vi "myFFT_RowSave.vi"(0 "freqs rows":i32[][](array[numeric]), 1 "小注入模式":u8, 2 "响应模式":u8 max=20, 3 "注入(1号)端口类型":u8(ring) items=["单相", "三相αβ系", "三相同步系", "三相正负序"], 4 "dq同步来源":u8(ring) items=["1号A相", "2号A相"], 5 "index row":i32[](array[numeric]), 6 "采样结果簇":T1, 7 "可用pico数(仅用于模式100)":u16, 9 "f_tick":dbl, 11 "f_mes":i32, 12 "稳态工作点输入":cdb[][](array[numeric]), 13 "写表结果输入":dbl[][](array[numeric]), 14 "基波频率 f_fun":u32=50 min=1 max=100000) -> (10 "稳态工作点输出":cdb[][](array[numeric]), 15 "写表结果输出":dbl[][](array[numeric]))   [LabVIEW 2024]
doc: "对于每个注入循环节，提取出FFT结果中的有效信息，存入稳态寄存器或输出结果寄存器。"
uses:
  <vilib>/Analysis/2dsp.llb/Real FFT.vi
  <vilib>/Analysis/NI_AALPro.lvlib
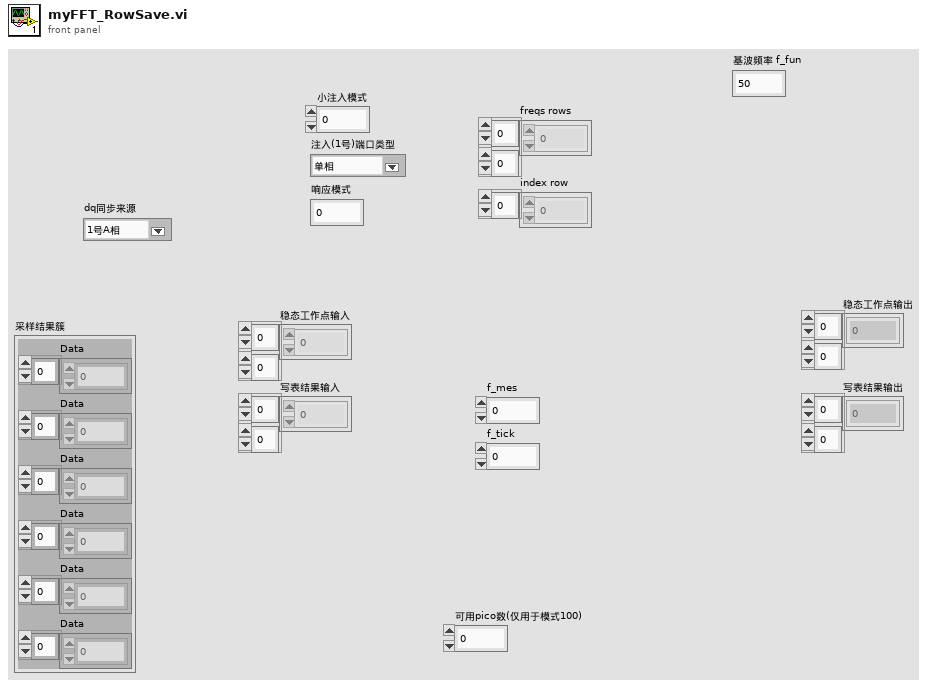
[diagram p1: front panel]
types:
  T1 = cluster{"Data":dbl[], "Data":dbl[], "Data":dbl[], "Data":dbl[], "Data":dbl[], "Data":dbl[]}
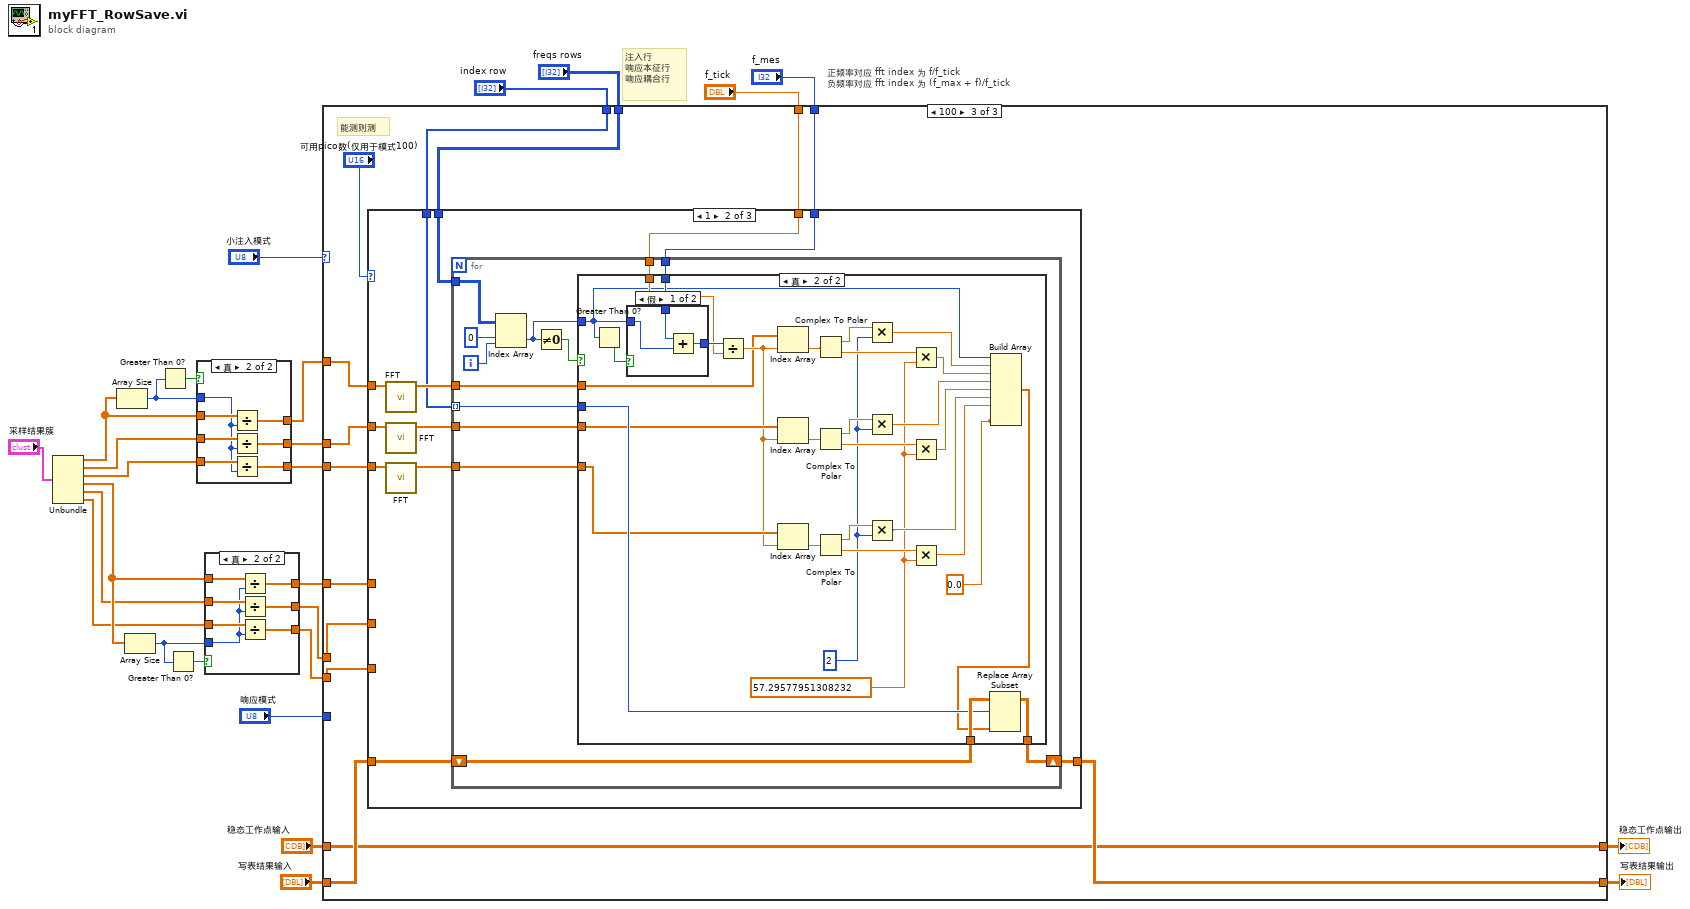
[diagram p0: block diagram]
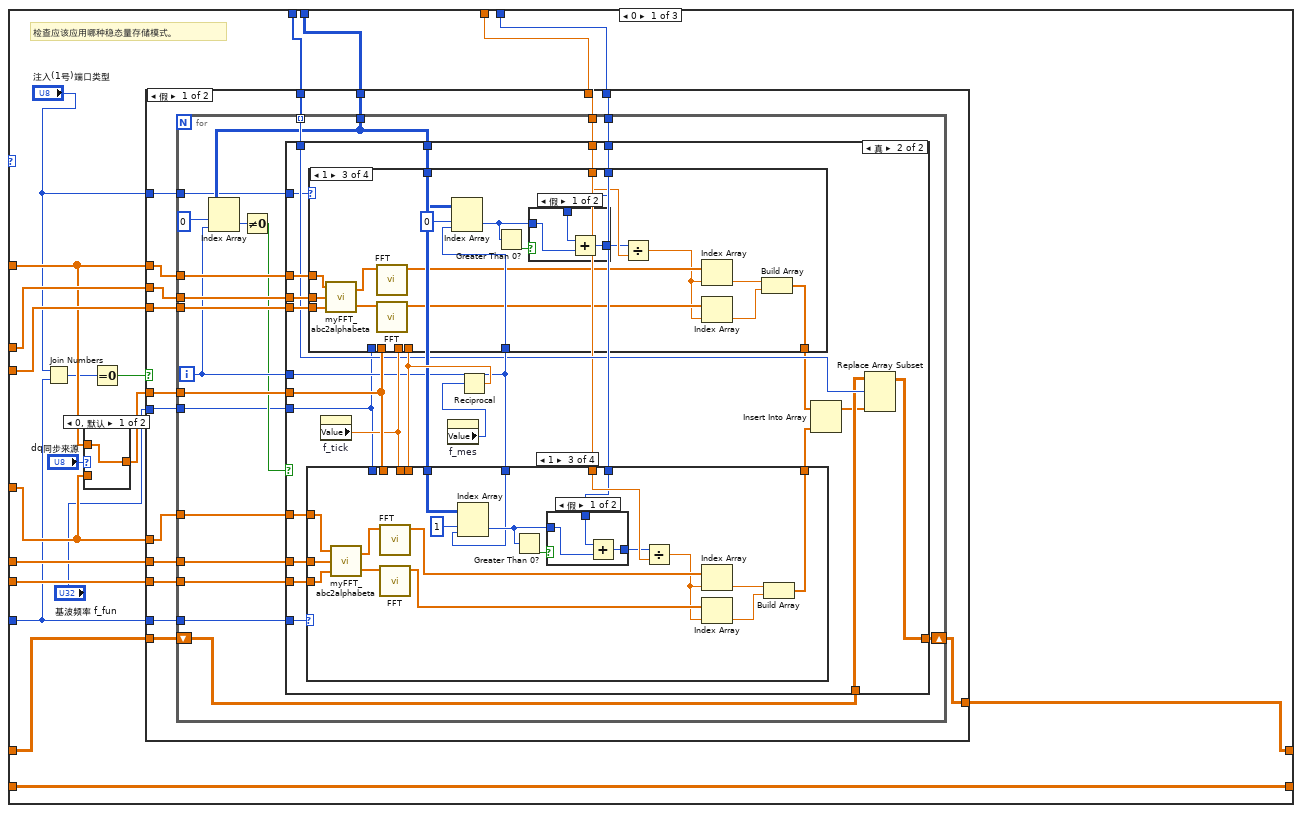
[diagram p4: hidden frame]
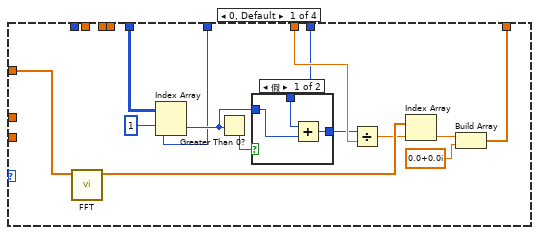
[diagram p7: hidden frame]
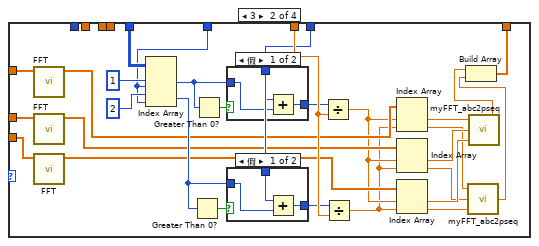
[diagram p9: hidden frame]
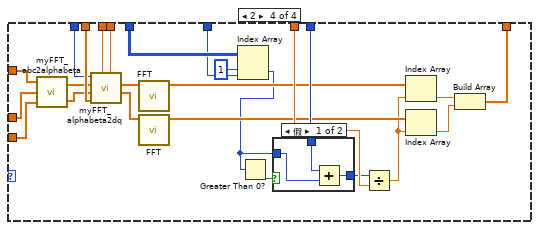
[diagram p13: hidden frame]
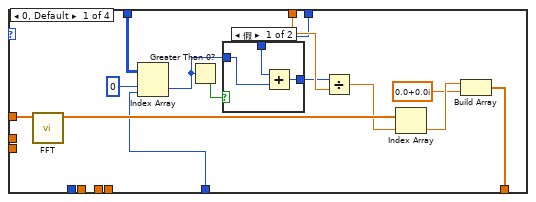
[diagram p15: hidden frame]
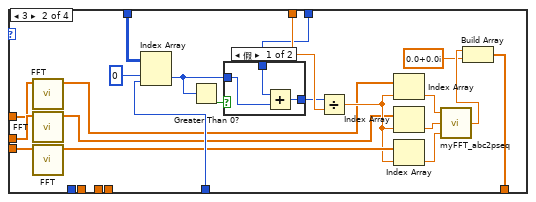
[diagram p17: hidden frame]
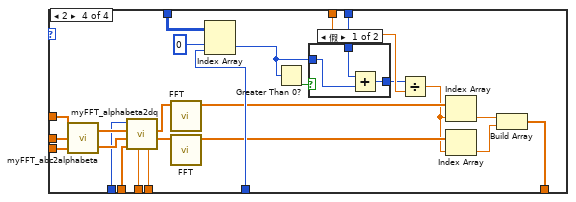
[diagram p20: hidden frame]
diagram:
  # "注入行\n响应本征行\n响应耦合行"
  # "正频率对应 fft index 为 f/f_tick\n负频率对应 fft index 为 (f_max + f)/f_tick"
  n1 = Unbundle("采样结果簇") -> ("Data"=w13:dbl[], "Data"=w11:dbl[], "Data"=w10:dbl[], "Data"=w6:dbl[], "Data"=w5:dbl[], "Data"=w4:dbl[])
  n2 = Array Size(array=w13) -> (size(s)=w16:i32)
  n3 = Array Size(array=w6) -> (size(s)=w7:i32)
  n4 = Greater Than 0?(x=w16) -> (x > 0?=w15:bool)
  n5 = Greater Than 0?(x=w7) -> (x > 0?=w8:bool)
  n6 = case shown="真" w15 {
    tunnel: w16 -> [_ w31]
    tunnel: [w28 w36] -> w14
    tunnel: w13 -> [w28 w37]
    tunnel: [w29 w35] -> w9
    tunnel: [w30 w34] -> w12
    tunnel: w10 -> [w29 w33]
    tunnel: w11 -> [w30 w32]
    frame False {
    }
    frame True {
      n7 = Divide(x=w37, y=w31) -> (x/y=w36:dbl[])
      n8 = Divide(x=w32, y=w31) -> (x/y=w34:dbl[])
      n9 = Divide(x=w33, y=w31) -> (x/y=w35:dbl[])
    }
  }
  n10 = case shown="真" w8 {
    tunnel: w7 -> [_ w41]
    tunnel: [w38 w46] -> w3
    tunnel: w6 -> [w38 w47]
    tunnel: [w39 w45] -> w1
    tunnel: [w40 w44] -> w2
    tunnel: w4 -> [w39 w43]
    tunnel: w5 -> [w40 w42]
    frame False {
    }
    frame True {
      n11 = Divide(x=w47, y=w41) -> (x/y=w46:dbl[])
      n12 = Divide(x=w42, y=w41) -> (x/y=w44:dbl[])
      n13 = Divide(x=w43, y=w41) -> (x/y=w45:dbl[])
    }
  }
  n14 = case shown="100" "小注入模式" {
    tunnel: "写表结果输入" -> [w67 w396 w869]
    tunnel: [w67 w395 w868] -> w24
    tunnel: "稳态工作点输入" -> [w58 w394 w867]
    tunnel: [w54 w394 w867] -> w25
    tunnel: w14 -> [w56 w399 w865]
    tunnel: w12 -> [w62 w404 w864]
    tunnel: w9 -> [w61 w403 w863]
    tunnel: w3 -> [w57 w400 w862]
    tunnel: w2 -> [w60 w402 w861]
    tunnel: w1 -> [w59 w401 w860]
    tunnel: "响应模式" -> [w51 w392 _]
    tunnel: "freqs rows" -> [w64 w406 w857]
    tunnel: "f_tick" -> [w65 w407 w859]
    tunnel: "f_mes" -> [w66 w408 w858]
    tunnel: "index row" -> [w63 w405 w856]
    frame 0 {
      # "检查应该应用哪种稳态量存储模式。"
      n15 = Join Numbers(hi="注入(1号)端口类型", lo=w51) -> ((hi.lo)=w50:u16)
      n16 = case shown="0, 默认" "dq同步来源" {
        tunnel: w56 -> [w68 _]
        tunnel: w57 -> [_ w69]
        tunnel: [w68 w69] -> w55
        frame 0, Default {
        }
        frame 1 {
        }
      }
      n17 = Equal To 0?(x=w50) -> (x = 0?=w49:bool)
      n18 = case shown="假" w49 {
        tunnel: w61 -> [w78 w335]
        tunnel: w56 -> [w81 w343]
        tunnel: "注入(1号)端口类型" -> [w70 _]
        tunnel: w51 -> [w73 _]
        tunnel: w57 -> [w77 _]
        tunnel: w60 -> [w76 _]
        tunnel: w59 -> [w75 _]
        tunnel: w62 -> [w79 w342]
        tunnel: w64 -> [w84 w341]
        tunnel: w58 -> [w80 w338]
        tunnel: w63 -> [w85 w337]
        tunnel: [w71 w336] -> w54
        tunnel: w65 -> [w83 w340]
        tunnel: w66 -> [w82 w339]
        tunnel: w55 -> [w74 _]
        tunnel: "基波频率 f_fun" -> [w72 _]
        frame False {
          n19 = for {
            tunnel: w85 -> [w95] mode=indexing
            tunnel: w84 -> [w91]
            tunnel: w83 -> [w98]
            tunnel: w82 -> [w97]
            tunnel: w81 -> [w105]
            shift-right: [w94] -> w71
            shift-left: w80 -> [w87]
            tunnel: w79 -> [w104]
            tunnel: w78 -> [w103]
            tunnel: w77 -> [w102]
            tunnel: w76 -> [w101]
            tunnel: w75 -> [w100]
            tunnel: w74 -> [w99]
            tunnel: w73 -> [w96]
            tunnel: w72 -> [w88]
            tunnel: w70 -> [w86]
            i -> [w92]
            n20 = Index Array(array=w91, index (row)=0 ("索引"), index (col)=w92) -> (element=w90:i32)
            n21 = Not Equal To 0?(x=w90) -> (x != 0?=w89:bool)
            n22 = case shown="真" w89 {
              tunnel: w105 -> [_ w129]
              tunnel: w104 -> [_ w128]
              tunnel: w103 -> [_ w127]
              tunnel: w102 -> [_ w126]
              tunnel: w101 -> [_ w125]
              tunnel: w100 -> [_ w124]
              tunnel: w99 -> [_ w123]
              tunnel: w91 -> [_ w119]
              tunnel: w98 -> [_ w108]
              tunnel: w97 -> [_ w118]
              tunnel: w92 -> [_ w117]
              tunnel: w96 -> [_ w116]
              tunnel: w95 -> [_ w115]
              tunnel: w87 -> [w106 w114]
              tunnel: [w106 w113] -> w94
              tunnel: w88 -> [_ w109]
              tunnel: w86 -> [_ w107]
              frame False {
              }
              frame True {
                n23 = property on="f_tick" class="DigNum (严格)"() -> ("Value"=w120:dbl)  [unwired: 2 in, 2 out]
                n24 = property on="f_mes" class="DigNum (严格)"() -> ("Value"=w122:i32)  [unwired: 2 in, 2 out]
                n25 = Reciprocal(x=w122) -> (1/x=w121:dbl)
                n26 = case shown="1" w116 {
                  tunnel: w121 -> [_ _ _ w232]
                  tunnel: w120 -> [_ _ _ w231]
                  tunnel: w123 -> [_ _ _ w230]
                  tunnel: w124 -> [_ w171 w200 w227]
                  tunnel: w125 -> [_ w173 w201 w226]
                  tunnel: w126 -> [w140 w174 w202 w225]
                  tunnel: w119 -> [w143 w172 w199 w223]
                  tunnel: w108 -> [w142 w176 w198 w222]
                  tunnel: w118 -> [w141 w175 w197 w221]
                  tunnel: w117 -> [w137 w148 w193 w218]
                  tunnel: [w135 w163 w190 w215] -> w111
                  tunnel: w109 -> [_ _ _ w209]
                  frame 0, Default {
                    n27 = call-poly <vilib>:"FFT.vi"("X"=w140) -> ("FFT {X}"=w136:cdb[])  [unwired: 9 in, 1 out]
                    n28 = Index Array(array=w143, index (row)=1 ("索引"), index (col)=w137) -> (element=w138:i32)
                    n29 = Greater Than 0?(x=w138) -> (x > 0?=w134:bool)
                    n30 = case shown="假" w134 {
                      tunnel: w138 -> [w145 w147]
                      tunnel: w141 -> [w146 _]
                      tunnel: [w144 w147] -> w133
                      frame False {
                        n31 = Add(x=w146, y=w145) -> (x+y=w144:i32)
                      }
                      frame True {
                      }
                    }
                    n32 = Divide(x=w133, y=w142) -> (x/y=w132:dbl)
                    n33 = Index Array(array=w136, index=w132) -> (element=w131:cdb)
                    n34 = Build Array(w131, cdb 0.0+0.0i ("元素")) -> (w135:cdb[])
                  }
                  frame 3 {
                    n35 = call-poly <vilib>:"FFT.vi"("X"=w174) -> ("FFT {X}"=w166:cdb[])  [unwired: 9 in, 1 out]
                    n36 = call-poly <vilib>:"FFT.vi"("X"=w173) -> ("FFT {X}"=w165:cdb[])  [unwired: 9 in, 1 out]
                    n37 = call-poly <vilib>:"FFT.vi"("X"=w171) -> ("FFT {X}"=w164:cdb[])  [unwired: 9 in, 1 out]
                    n38 = Index Array(array=w172, index (row) #1=1 ("索引"), index (col) #1=w148, index (row) #2=2 ("索引 (行)"), index (col) #2=w148) -> (element #1=w169:i32, element #2=w167:i32)
                    n39 = Greater Than 0?(x=w167) -> (x > 0?=w156:bool)
                    n40 = Greater Than 0?(x=w169) -> (x > 0?=w162:bool)
                    n41 = case shown="假" w162 {
                      tunnel: w169 -> [w182 w184]
                      tunnel: w175 -> [w183 _]
                      tunnel: [w181 w184] -> w161
                      frame False {
                        n42 = Add(x=w183, y=w182) -> (x+y=w181:i32)
                      }
                      frame True {
                      }
                    }
                    n43 = case shown="假" w156 {
                      tunnel: w167 -> [w178 w180]
                      tunnel: w175 -> [w179 _]
                      tunnel: [w177 w180] -> w155
                      frame False {
                        n44 = Add(x=w179, y=w178) -> (x+y=w177:i32)
                      }
                      frame True {
                      }
                    }
                    n45 = Divide(x=w161, y=w176) -> (x/y=w160:dbl)
                    n46 = Divide(x=w155, y=w176) -> (x/y=w154:dbl)
                    n47 = Index Array(array=w166, index #1=w160, index #2=w154) -> (element #1=w159:cdb, element #2=w153:cdb)
                    n48 = Index Array(array=w165, index #1=w160, index #2=w154) -> (element #1=w158:cdb, element #2=w152:cdb)
                    n49 = Index Array(array=w164, index #1=w160, index #2=w154) -> (element #1=w157:cdb, element #2=w151:cdb)
                    n50 = call "myFFT_abc2pseq.vi"("C spec"=w151, "B spec"=w152, "A spec"=w153) -> ("p seq spec"=w149:cdb)
                    n51 = call "myFFT_abc2pseq.vi"("C spec"=w157, "B spec"=w158, "A spec"=w159) -> ("p seq spec"=w150:cdb)
                    n52 = Build Array(w150, w149) -> (w163:cdb[])
                  }
                  frame 1 {
                    n53 = call "myFFT_abc2alphabeta.vi"("C wave"=w200, "B wave"=w201, "A wave"=w202) -> ("beta wave"=w196:dbl[], "alpha wave"=w203:dbl[])
                    n54 = call-poly <vilib>:"FFT.vi"("X"=w203) -> ("FFT {X}"=w192:cdb[])  [unwired: 9 in, 1 out]
                    n55 = call-poly <vilib>:"FFT.vi"("X"=w196) -> ("FFT {X}"=w191:cdb[])  [unwired: 9 in, 1 out]
                    n56 = Index Array(array=w199, index (row)=1 ("索引"), index (col)=w193) -> (element=w194:i32)
                    n57 = Greater Than 0?(x=w194) -> (x > 0?=w189:bool)
                    n58 = case shown="假" w189 {
                      tunnel: w194 -> [w205 w207]
                      tunnel: w197 -> [w206 _]
                      tunnel: [w204 w207] -> w188
                      frame False {
                        n59 = Add(x=w206, y=w205) -> (x+y=w204:i32)
                      }
                      frame True {
                      }
                    }
                    n60 = Divide(x=w188, y=w198) -> (x/y=w187:dbl)
                    n61 = Index Array(array=w192, index=w187) -> (element=w186:cdb)
                    n62 = Index Array(array=w191, index=w187) -> (element=w185:cdb)
                    n63 = Build Array(w186, w185) -> (w190:cdb[])
                  }
                  frame 2 {
                    n64 = call "myFFT_abc2alphabeta.vi"("C wave"=w227, "B wave"=w226, "A wave"=w225) -> ("beta wave"=w228:dbl[], "alpha wave"=w229:dbl[])
                    n65 = call "myFFT_alphabeta2dq.vi"("t_tick"=w232, "f_tick"=w231, "ref wave"=w230, "beta wave"=w228, "alpha wave"=w229, "基波频率"=w209) -> ("q wave"=w220:dbl[], "d wave"=w224:dbl[])  [unwired: 4 in]
                    n66 = call-poly <vilib>:"FFT.vi"("X"=w224) -> ("FFT {X}"=w217:cdb[])  [unwired: 9 in, 1 out]
                    n67 = call-poly <vilib>:"FFT.vi"("X"=w220) -> ("FFT {X}"=w216:cdb[])  [unwired: 9 in, 1 out]
                    n68 = Index Array(array=w223, index (row)=1 ("索引"), index (col)=w218) -> (element=w208:i32)
                    n69 = Greater Than 0?(x=w208) -> (x > 0?=w214:bool)
                    n70 = case shown="假" w214 {
                      tunnel: w208 -> [w234 w236]
                      tunnel: w221 -> [w235 _]
                      tunnel: [w233 w236] -> w213
                      frame False {
                        n71 = Add(x=w235, y=w234) -> (x+y=w233:i32)
                      }
                      frame True {
                      }
                    }
                    n72 = Divide(x=w213, y=w222) -> (x/y=w212:dbl)
                    n73 = Index Array(array=w217, index=w212) -> (element=w211:cdb)
                    n74 = Index Array(array=w216, index=w212) -> (element=w210:cdb)
                    n75 = Build Array(w211, w210) -> (w215:cdb[])
                  }
                }
                n76 = case shown="1" w107 {
                  tunnel: w121 -> [_ _ _ w327]
                  tunnel: w120 -> [_ _ _ w326]
                  tunnel: w123 -> [_ _ _ w325]
                  tunnel: w129 -> [w246 w271 w298 w322]
                  tunnel: w119 -> [w250 w275 w293 w318]
                  tunnel: w108 -> [w249 w274 w295 w317]
                  tunnel: w118 -> [w248 w255 w294 w316]
                  tunnel: w128 -> [_ w272 w297 w321]
                  tunnel: w127 -> [_ w273 w296 w320]
                  tunnel: w117 -> [w243 w268 w288 w312]
                  tunnel: [w242 w266 w285 w309] -> w112
                  tunnel: w109 -> [_ _ _ w303]
                  frame 0, Default {
                    n77 = call-poly <vilib>:"FFT.vi"("X"=w246) -> ("FFT {X}"=w247:cdb[])  [unwired: 9 in, 1 out]
                    n78 = Index Array(array=w250, index (row)=0 ("索引"), index (col)=w243) -> (element=w244:i32)
                    n79 = Greater Than 0?(x=w244) -> (x > 0?=w241:bool)
                    n80 = case shown="假" w241 {
                      tunnel: w244 -> [w252 w254]
                      tunnel: w248 -> [w253 _]
                      tunnel: [w251 w254] -> w240
                      frame False {
                        n81 = Add(x=w253, y=w252) -> (x+y=w251:i32)
                      }
                      frame True {
                      }
                    }
                    n82 = Divide(x=w240, y=w249) -> (x/y=w239:dbl)
                    n83 = Index Array(array=w247, index=w239) -> (element=w238:cdb)
                    n84 = Build Array(w238, cdb 0.0+0.0i ("元素")) -> (w242:cdb[])
                  }
                  frame 3 {
                    n85 = call-poly <vilib>:"FFT.vi"("X"=w271) -> ("FFT {X}"=w256:cdb[])  [unwired: 9 in, 1 out]
                    n86 = call-poly <vilib>:"FFT.vi"("X"=w272) -> ("FFT {X}"=w257:cdb[])  [unwired: 9 in, 1 out]
                    n87 = call-poly <vilib>:"FFT.vi"("X"=w273) -> ("FFT {X}"=w267:cdb[])  [unwired: 9 in, 1 out]
                    n88 = Index Array(array=w275, index (row)=0 ("索引"), index (col)=w268) -> (element=w269:i32)
                    n89 = Greater Than 0?(x=w269) -> (x > 0?=w265:bool)
                    n90 = case shown="假" w265 {
                      tunnel: w269 -> [w277 w279]
                      tunnel: w255 -> [w278 _]
                      tunnel: [w276 w279] -> w264
                      frame False {
                        n91 = Add(x=w278, y=w277) -> (x+y=w276:i32)
                      }
                      frame True {
                      }
                    }
                    n92 = Divide(x=w264, y=w274) -> (x/y=w263:dbl)
                    n93 = Index Array(array=w256, index=w263) -> (element=w262:cdb)
                    n94 = Index Array(array=w257, index=w263) -> (element=w261:cdb)
                    n95 = Index Array(array=w267, index=w263) -> (element=w260:cdb)
                    n96 = call "myFFT_abc2pseq.vi"("C spec"=w260, "B spec"=w261, "A spec"=w262) -> ("p seq spec"=w259:cdb)
                    n97 = Build Array(w259, cdb 0.0+0.0i ("元素")) -> (w266:cdb[])
                  }
                  frame 1 {
                    n98 = call "myFFT_abc2alphabeta.vi"("C wave"=w296, "B wave"=w297, "A wave"=w298) -> ("beta wave"=w292:dbl[], "alpha wave"=w291:dbl[])
                    n99 = call-poly <vilib>:"FFT.vi"("X"=w291) -> ("FFT {X}"=w287:cdb[])  [unwired: 9 in, 1 out]
                    n100 = call-poly <vilib>:"FFT.vi"("X"=w292) -> ("FFT {X}"=w286:cdb[])  [unwired: 9 in, 1 out]
                    n101 = Index Array(array=w293, index (row)=0 ("索引"), index (col)=w288) -> (element=w289:i32)
                    n102 = Greater Than 0?(x=w289) -> (x > 0?=w284:bool)
                    n103 = case shown="假" w284 {
                      tunnel: w289 -> [w300 w302]
                      tunnel: w294 -> [w301 _]
                      tunnel: [w299 w302] -> w283
                      frame False {
                        n104 = Add(x=w301, y=w300) -> (x+y=w299:i32)
                      }
                      frame True {
                      }
                    }
                    n105 = Divide(x=w283, y=w295) -> (x/y=w282:dbl)
                    n106 = Index Array(array=w287, index=w282) -> (element=w281:cdb)
                    n107 = Index Array(array=w286, index=w282) -> (element=w280:cdb)
                    n108 = Build Array(w281, w280) -> (w285:cdb[])
                  }
                  frame 2 {
                    n109 = call "myFFT_abc2alphabeta.vi"("C wave"=w320, "B wave"=w321, "A wave"=w322) -> ("beta wave"=w323:dbl[], "alpha wave"=w324:dbl[])
                    n110 = call "myFFT_alphabeta2dq.vi"("t_tick"=w327, "f_tick"=w326, "ref wave"=w325, "beta wave"=w323, "alpha wave"=w324, "基波频率"=w303) -> ("q wave"=w319:dbl[], "d wave"=w315:dbl[])  [unwired: 4 in]
                    n111 = call-poly <vilib>:"FFT.vi"("X"=w315) -> ("FFT {X}"=w311:cdb[])  [unwired: 9 in, 1 out]
                    n112 = call-poly <vilib>:"FFT.vi"("X"=w319) -> ("FFT {X}"=w310:cdb[])  [unwired: 9 in, 1 out]
                    n113 = Index Array(array=w318, index (row)=0 ("索引"), index (col)=w312) -> (element=w313:i32)
                    n114 = Greater Than 0?(x=w313) -> (x > 0?=w308:bool)
                    n115 = case shown="假" w308 {
                      tunnel: w313 -> [w329 w331]
                      tunnel: w316 -> [w330 _]
                      tunnel: [w328 w331] -> w307
                      frame False {
                        n116 = Add(x=w330, y=w329) -> (x+y=w328:i32)
                      }
                      frame True {
                      }
                    }
                    n117 = Divide(x=w307, y=w317) -> (x/y=w306:dbl)
                    n118 = Index Array(array=w311, index=w306) -> (element=w305:cdb)
                    n119 = Index Array(array=w310, index=w306) -> (element=w304:cdb)
                    n120 = Build Array(w305, w304) -> (w309:cdb[])
                  }
                }
                n121 = Insert Into Array(array=w112, new element=w111) -> (w110:cdb[])  [unwired: 1 in]
                n122 = Replace Array Subset(array=w114, new element=w110, index (row)=w115) -> (w113:cdb[][])  [unwired: 1 in]
              }
            }
          }
        }
        frame True {
          n123 = call-poly <vilib>:"FFT.vi"("X"=w343) -> ("FFT {X}"=w334:cdb[])  [unwired: 9 in, 1 out]
          n124 = call-poly <vilib>:"FFT.vi"("X"=w342) -> ("FFT {X}"=w333:cdb[])  [unwired: 9 in, 1 out]
          n125 = call-poly <vilib>:"FFT.vi"("X"=w335) -> ("FFT {X}"=w332:cdb[])  [unwired: 9 in, 1 out]
          n126 = for {
            tunnel: w341 -> [w358]
            tunnel: w340 -> [w352]
            tunnel: w339 -> [w351]
            tunnel: w334 -> [w349]
            tunnel: w333 -> [w348]
            tunnel: w332 -> [w347]
            shift-right: [w344] -> w336
            shift-left: w338 -> [w346]
            tunnel: w337 -> [w345] mode=indexing
            i -> [w357]
            n127 = Index Array(array=w358, index (row) #1=0 ("索引"), index (col) #1=w357, index (row) #2=1 ("索引"), index (col) #2=w357) -> (element #1=w353:i32, element #2=w350:i32)
            n128 = Not Equal To 0?(x=w353) -> (x != 0?=w354:bool)
            n129 = case shown="真" w354 {
              tunnel: w353 -> [_ w379]
              tunnel: w352 -> [_ w374]
              tunnel: w351 -> [_ w375]
              tunnel: w350 -> [_ w376]
              tunnel: w349 -> [_ w372]
              tunnel: w348 -> [_ w371]
              tunnel: w347 -> [_ w370]
              tunnel: w346 -> [w359 w365]
              tunnel: w345 -> [_ w364]
              tunnel: [w359 w363] -> w344
              frame False {
              }
              frame True {
                n130 = Greater Than 0?(x=w376) -> (x > 0?=w377:bool)
                n131 = Greater Than 0?(x=w379) -> (x > 0?=w380:bool)
                n132 = case shown="假" w380 {
                  tunnel: w379 -> [w386 w388]
                  tunnel: w375 -> [w387 _]
                  tunnel: [w385 w388] -> w378
                  frame False {
                    n133 = Add(x=w387, y=w386) -> (x+y=w385:i32)
                  }
                  frame True {
                  }
                }
                n134 = case shown="假" w377 {
                  tunnel: w376 -> [w382 w384]
                  tunnel: w375 -> [w383 _]
                  tunnel: [w381 w384] -> w373
                  frame False {
                    n135 = Add(x=w383, y=w382) -> (x+y=w381:i32)
                  }
                  frame True {
                  }
                }
                n136 = Divide(x=w378, y=w374) -> (x/y=w369:dbl)
                n137 = Divide(x=w373, y=w374) -> (x/y=w368:dbl)
                n138 = Index Array(array=w372, index=w369) -> (element=w367:cdb)
                n139 = Index Array(array=w371, index=w368) -> (element=w362:cdb)
                n140 = Index Array(array=w370, index=w368) -> (element=w361:cdb)
                n141 = Build Array(w367, cdb 0.0+0.0i ("元素"), w362, w361) -> (w366:cdb[])
                n142 = Replace Array Subset(array=w365, new element=w366, index (row)=w364) -> (w363:cdb[][])  [unwired: 1 in]
              }
            }
          }
        }
      }
    }
    frame 1, Default {
      # "注入-响应 在小信号测量情况下。在此情况下，对注入输出模式分别做判断。"
      n143 = property on="注入(1号)端口类型" class="Ring (严格)"() -> ("Value"=w393:u8)  [unwired: 2 in, 2 out]
      n144 = Join Numbers(hi=w393, lo=w392) -> ((hi.lo)=w391:u16)
      n145 = property on="dq同步来源" class="Ring (严格)"() -> ("Value"=w389:u8)  [unwired: 2 in, 2 out]
      n146 = property on="基波频率 f_fun" class="DigNum (严格)"() -> ("Value"=w397:u32)  [unwired: 2 in, 2 out]
      n147 = case shown="0, 默认" w389 {
        tunnel: w399 -> [w409 _]
        tunnel: w400 -> [_ w410]
        tunnel: [w409 w410] -> w398
        frame 0, Default {
        }
        frame 1 {
        }
      }
      n148 = Equal To 0?(x=w391) -> (x = 0?=w390:bool)
      n149 = case shown="假" w390 {
        tunnel: w403 -> [w420 w782]
        tunnel: w399 -> [w423 w790]
        tunnel: w393 -> [w412 _]
        tunnel: w392 -> [w415 _]
        tunnel: w400 -> [w419 _]
        tunnel: w402 -> [w418 _]
        tunnel: w401 -> [w417 _]
        tunnel: w404 -> [w421 w789]
        tunnel: w406 -> [w426 w788]
        tunnel: w396 -> [w422 w785]
        tunnel: w405 -> [w427 w784]
        tunnel: [w413 w783] -> w395
        tunnel: w407 -> [w425 w787]
        tunnel: w408 -> [w424 w786]
        tunnel: w398 -> [w416 _]
        tunnel: w397 -> [w414 _]
        tunnel: w394 -> [w411 w778]
        frame False {
          n150 = for {
            tunnel: w427 -> [w439] mode=indexing
            tunnel: w426 -> [w436]
            tunnel: w425 -> [w442]
            tunnel: w424 -> [w441]
            tunnel: w423 -> [w449]
            shift-right: [w438] -> w413
            shift-left: w422 -> [w431]
            tunnel: w421 -> [w448]
            tunnel: w420 -> [w447]
            tunnel: w419 -> [w446]
            tunnel: w418 -> [w445]
            tunnel: w417 -> [w444]
            tunnel: w416 -> [w443]
            tunnel: w415 -> [w440]
            tunnel: w414 -> [w433]
            tunnel: w412 -> [w432]
            tunnel: w411 -> [w430]
            i -> [w428]
            n151 = Index Array(array=w436, index (row)=0 ("索引"), index (col)=w428) -> (element=w435:i32)
            n152 = Index Array(array=w430, index (row)=w428) -> (element=w429:cdb[])  [unwired: 1 in]
            n153 = Not Equal To 0?(x=w435) -> (x != 0?=w434:bool)
            n154 = case shown="真" w434 {
              tunnel: w449 -> [_ w488]
              tunnel: w448 -> [_ w487]
              tunnel: w447 -> [_ w486]
              tunnel: w446 -> [_ w485]
              tunnel: w445 -> [_ w484]
              tunnel: w444 -> [_ w483]
              tunnel: w443 -> [_ w482]
              tunnel: w436 -> [_ w451]
              tunnel: w442 -> [_ w474]
              tunnel: w441 -> [_ w478]
              tunnel: w428 -> [_ w453]
              tunnel: w440 -> [_ w477]
              tunnel: w439 -> [_ w462]
              tunnel: [w450 w476] -> w438
              tunnel: w433 -> [_ w475]
              tunnel: w432 -> [_ w473]
              tunnel: w431 -> [w450 w472]
              tunnel: w429 -> [_ w471]
              frame False {
              }
              frame True {
                n155 = property on="f_tick" class="DigNum (严格)"() -> ("Value"=w479:dbl)  [unwired: 2 in, 2 out]
                n156 = property on="f_mes" class="DigNum (严格)"() -> ("Value"=w481:i32)  [unwired: 2 in, 2 out]
                n157 = Reciprocal(x=w481) -> (1/x=w480:dbl)
                n158 = Index Array(array=w471, index #1=0 ("索引"), index #2=1 ("索引"), index #3=2 ("索引"), index #4=3 ("索引")) -> (element #1=w466:cdb, element #2=w465:cdb, element #3=w464:cdb, element #4=w463:cdb)
                n159 = case shown="0, 默认" w477 {
                  tunnel: w480 -> [_ _ _ w670]
                  tunnel: w479 -> [_ _ _ w669]
                  tunnel: w482 -> [_ _ _ w668]
                  tunnel: w483 -> [_ w603 w635 w665]
                  tunnel: w484 -> [_ w605 w636 w664]
                  tunnel: w485 -> [w569 w606 w637 w663]
                  tunnel: w451 -> [w572 w604 w634 w661]
                  tunnel: w474 -> [w571 w608 w633 w660]
                  tunnel: w478 -> [w570 w607 w632 w659]
                  tunnel: w453 -> [w566 w583 w628 w656]
                  tunnel: w475 -> [_ _ _ w650]
                  tunnel: w464 -> [w560 w581 w620 w646]
                  tunnel: w463 -> [_ w577 w619 w645]
                  tunnel: [w559 w578 w618 w643] -> w459
                  tunnel: [cdb 0.0+0.0i ("元素") w579 w617 w644] -> w458
                  frame 0, Default {
                    n160 = call-poly <vilib>:"FFT.vi"("X"=w569) -> ("FFT {X}"=w565:cdb[])  [unwired: 9 in, 1 out]
                    n161 = Index Array(array=w572, index (row)=1 ("索引"), index (col)=w566) -> (element=w567:i32)
                    n162 = Greater Than 0?(x=w567) -> (x > 0?=w564:bool)
                    n163 = case shown="假" w564 {
                      tunnel: w567 -> [w574 w576]
                      tunnel: w570 -> [w575 _]
                      tunnel: [w573 w576] -> w563
                      frame False {
                        n164 = Add(x=w575, y=w574) -> (x+y=w573:i32)
                      }
                      frame True {
                      }
                    }
                    n165 = Divide(x=w563, y=w571) -> (x/y=w562:dbl)
                    n166 = Index Array(array=w565, index=w562) -> (element=w561:cdb)
                    n167 = Subtract(x=w561, y=w560) -> (x-y=w559:cdb)
                  }
                  frame 3 {
                    n168 = call-poly <vilib>:"FFT.vi"("X"=w606) -> ("FFT {X}"=w598:cdb[])  [unwired: 9 in, 1 out]
                    n169 = call-poly <vilib>:"FFT.vi"("X"=w605) -> ("FFT {X}"=w597:cdb[])  [unwired: 9 in, 1 out]
                    n170 = call-poly <vilib>:"FFT.vi"("X"=w603) -> ("FFT {X}"=w596:cdb[])  [unwired: 9 in, 1 out]
                    n171 = Index Array(array=w604, index (row) #1=1 ("索引"), index (col) #1=w583, index (row) #2=2 ("索引 (行)"), index (col) #2=w583) -> (element #1=w601:i32, element #2=w599:i32)
                    n172 = Greater Than 0?(x=w599) -> (x > 0?=w589:bool)
                    n173 = Greater Than 0?(x=w601) -> (x > 0?=w595:bool)
                    n174 = case shown="假" w595 {
                      tunnel: w601 -> [w614 w616]
                      tunnel: w607 -> [w615 _]
                      tunnel: [w613 w616] -> w594
                      frame False {
                        n175 = Add(x=w615, y=w614) -> (x+y=w613:i32)
                      }
                      frame True {
                      }
                    }
                    n176 = case shown="假" w589 {
                      tunnel: w599 -> [w610 w612]
                      tunnel: w607 -> [w611 _]
                      tunnel: [w609 w612] -> w588
                      frame False {
                        n177 = Add(x=w611, y=w610) -> (x+y=w609:i32)
                      }
                      frame True {
                      }
                    }
                    n178 = Divide(x=w594, y=w608) -> (x/y=w593:dbl)
                    n179 = Divide(x=w588, y=w608) -> (x/y=w587:dbl)
                    n180 = Index Array(array=w598, index #1=w593, index #2=w587) -> (element #1=w592:cdb, element #2=w586:cdb)
                    n181 = Index Array(array=w597, index #1=w593, index #2=w587) -> (element #1=w591:cdb, element #2=w585:cdb)
                    n182 = Index Array(array=w596, index #1=w593, index #2=w587) -> (element #1=w590:cdb, element #2=w584:cdb)
                    n183 = call "myFFT_abc2pseq.vi"("C spec"=w584, "B spec"=w585, "A spec"=w586) -> ("p seq spec"=w580:cdb)
                    n184 = call "myFFT_abc2pseq.vi"("C spec"=w590, "B spec"=w591, "A spec"=w592) -> ("p seq spec"=w582:cdb)
                    n185 = Subtract(x=w582, y=w581) -> (x-y=w578:cdb)
                    n186 = Subtract(x=w580, y=w577) -> (x-y=w579:cdb)
                  }
                  frame 1 {
                    n187 = call "myFFT_abc2alphabeta.vi"("C wave"=w635, "B wave"=w636, "A wave"=w637) -> ("beta wave"=w631:dbl[], "alpha wave"=w638:dbl[])
                    n188 = call-poly <vilib>:"FFT.vi"("X"=w638) -> ("FFT {X}"=w627:cdb[])  [unwired: 9 in, 1 out]
                    n189 = call-poly <vilib>:"FFT.vi"("X"=w631) -> ("FFT {X}"=w626:cdb[])  [unwired: 9 in, 1 out]
                    n190 = Index Array(array=w634, index (row)=1 ("索引"), index (col)=w628) -> (element=w629:i32)
                    n191 = Greater Than 0?(x=w629) -> (x > 0?=w625:bool)
                    n192 = case shown="假" w625 {
                      tunnel: w629 -> [w640 w642]
                      tunnel: w632 -> [w641 _]
                      tunnel: [w639 w642] -> w624
                      frame False {
                        n193 = Add(x=w641, y=w640) -> (x+y=w639:i32)
                      }
                      frame True {
                      }
                    }
                    n194 = Divide(x=w624, y=w633) -> (x/y=w623:dbl)
                    n195 = Index Array(array=w627, index=w623) -> (element=w622:cdb)
                    n196 = Index Array(array=w626, index=w623) -> (element=w621:cdb)
                    n197 = Subtract(x=w622, y=w620) -> (x-y=w618:cdb)
                    n198 = Subtract(x=w621, y=w619) -> (x-y=w617:cdb)
                  }
                  frame 2 {
                    n199 = call "myFFT_abc2alphabeta.vi"("C wave"=w665, "B wave"=w664, "A wave"=w663) -> ("beta wave"=w666:dbl[], "alpha wave"=w667:dbl[])
                    n200 = call "myFFT_alphabeta2dq.vi"("t_tick"=w670, "f_tick"=w669, "ref wave"=w668, "beta wave"=w666, "alpha wave"=w667, "基波频率"=w650) -> ("q wave"=w658:dbl[], "d wave"=w662:dbl[])  [unwired: 4 in]
                    n201 = call-poly <vilib>:"FFT.vi"("X"=w662) -> ("FFT {X}"=w655:cdb[])  [unwired: 9 in, 1 out]
                    n202 = call-poly <vilib>:"FFT.vi"("X"=w658) -> ("FFT {X}"=w654:cdb[])  [unwired: 9 in, 1 out]
                    n203 = Index Array(array=w661, index (row)=1 ("索引"), index (col)=w656) -> (element=w649:i32)
                    n204 = Greater Than 0?(x=w649) -> (x > 0?=w653:bool)
                    n205 = case shown="假" w653 {
                      tunnel: w649 -> [w672 w674]
                      tunnel: w659 -> [w673 _]
                      tunnel: [w671 w674] -> w652
                      frame False {
                        n206 = Add(x=w673, y=w672) -> (x+y=w671:i32)
                      }
                      frame True {
                      }
                    }
                    n207 = Divide(x=w652, y=w660) -> (x/y=w651:dbl)
                    n208 = Index Array(array=w655, index=w651) -> (element=w648:cdb)
                    n209 = Index Array(array=w654, index=w651) -> (element=w647:cdb)
                    n210 = Subtract(x=w648, y=w646) -> (x-y=w643:cdb)
                    n211 = Subtract(x=w647, y=w645) -> (x-y=w644:cdb)
                  }
                }
                n212 = case shown="2" w473 {
                  tunnel: w480 -> [_ _ _ w773]
                  tunnel: w479 -> [_ _ _ w772]
                  tunnel: w482 -> [_ _ _ w771]
                  tunnel: w488 -> [w685 w711 w741 w768]
                  tunnel: w451 -> [w689 w715 w736 w764]
                  tunnel: w474 -> [w688 w714 w738 w763]
                  tunnel: w478 -> [w687 w698 w737 w762]
                  tunnel: w487 -> [_ w712 w740 w767]
                  tunnel: w486 -> [_ w713 w739 w766]
                  tunnel: w453 -> [w682 w708 w731 w758]
                  tunnel: w475 -> [_ _ _ w752]
                  tunnel: w466 -> [w677 w696 w723 w748]
                  tunnel: w465 -> [_ _ w722 w749]
                  tunnel: [cdb 0.0+0.0i ("元素") cdb 0.0+0.0i ("元素") w721 w746] -> w461
                  tunnel: [w675 w695 w720 w747] -> w460
                  frame 0, Default {
                    n213 = call-poly <vilib>:"FFT.vi"("X"=w685) -> ("FFT {X}"=w686:cdb[])  [unwired: 9 in, 1 out]
                    n214 = Index Array(array=w689, index (row)=0 ("索引"), index (col)=w682) -> (element=w683:i32)
                    n215 = Greater Than 0?(x=w683) -> (x > 0?=w681:bool)
                    n216 = case shown="假" w681 {
                      tunnel: w683 -> [w691 w693]
                      tunnel: w687 -> [w692 _]
                      tunnel: [w690 w693] -> w680
                      frame False {
                        n217 = Add(x=w692, y=w691) -> (x+y=w690:i32)
                      }
                      frame True {
                      }
                    }
                    n218 = Divide(x=w680, y=w688) -> (x/y=w679:dbl)
                    n219 = Index Array(array=w686, index=w679) -> (element=w678:cdb)
                    n220 = Subtract(x=w678, y=w677) -> (x-y=w675:cdb)
                  }
                  frame 3 {
                    n221 = call-poly <vilib>:"FFT.vi"("X"=w711) -> ("FFT {X}"=w699:cdb[])  [unwired: 9 in, 1 out]
                    n222 = call-poly <vilib>:"FFT.vi"("X"=w712) -> ("FFT {X}"=w700:cdb[])  [unwired: 9 in, 1 out]
                    n223 = call-poly <vilib>:"FFT.vi"("X"=w713) -> ("FFT {X}"=w707:cdb[])  [unwired: 9 in, 1 out]
                    n224 = Index Array(array=w715, index (row)=0 ("索引"), index (col)=w708) -> (element=w709:i32)
                    n225 = Greater Than 0?(x=w709) -> (x > 0?=w706:bool)
                    n226 = case shown="假" w706 {
                      tunnel: w709 -> [w717 w719]
                      tunnel: w698 -> [w718 _]
                      tunnel: [w716 w719] -> w705
                      frame False {
                        n227 = Add(x=w718, y=w717) -> (x+y=w716:i32)
                      }
                      frame True {
                      }
                    }
                    n228 = Divide(x=w705, y=w714) -> (x/y=w704:dbl)
                    n229 = Index Array(array=w699, index=w704) -> (element=w703:cdb)
                    n230 = Index Array(array=w700, index=w704) -> (element=w702:cdb)
                    n231 = Index Array(array=w707, index=w704) -> (element=w701:cdb)
                    n232 = call "myFFT_abc2pseq.vi"("C spec"=w701, "B spec"=w702, "A spec"=w703) -> ("p seq spec"=w697:cdb)
                    n233 = Subtract(x=w697, y=w696) -> (x-y=w695:cdb)
                  }
                  frame 1 {
                    n234 = call "myFFT_abc2alphabeta.vi"("C wave"=w739, "B wave"=w740, "A wave"=w741) -> ("beta wave"=w735:dbl[], "alpha wave"=w734:dbl[])
                    n235 = call-poly <vilib>:"FFT.vi"("X"=w734) -> ("FFT {X}"=w730:cdb[])  [unwired: 9 in, 1 out]
                    n236 = call-poly <vilib>:"FFT.vi"("X"=w735) -> ("FFT {X}"=w729:cdb[])  [unwired: 9 in, 1 out]
                    n237 = Index Array(array=w736, index (row)=0 ("索引"), index (col)=w731) -> (element=w732:i32)
                    n238 = Greater Than 0?(x=w732) -> (x > 0?=w728:bool)
                    n239 = case shown="假" w728 {
                      tunnel: w732 -> [w743 w745]
                      tunnel: w737 -> [w744 _]
                      tunnel: [w742 w745] -> w727
                      frame False {
                        n240 = Add(x=w744, y=w743) -> (x+y=w742:i32)
                      }
                      frame True {
                      }
                    }
                    n241 = Divide(x=w727, y=w738) -> (x/y=w726:dbl)
                    n242 = Index Array(array=w730, index=w726) -> (element=w725:cdb)
                    n243 = Index Array(array=w729, index=w726) -> (element=w724:cdb)
                    n244 = Subtract(x=w725, y=w723) -> (x-y=w720:cdb)
                    n245 = Subtract(x=w724, y=w722) -> (x-y=w721:cdb)
                  }
                  frame 2 {
                    n246 = call "myFFT_abc2alphabeta.vi"("C wave"=w766, "B wave"=w767, "A wave"=w768) -> ("beta wave"=w769:dbl[], "alpha wave"=w770:dbl[])
                    n247 = call "myFFT_alphabeta2dq.vi"("t_tick"=w773, "f_tick"=w772, "ref wave"=w771, "beta wave"=w769, "alpha wave"=w770, "基波频率"=w752) -> ("q wave"=w765:dbl[], "d wave"=w761:dbl[])  [unwired: 4 in]
                    n248 = call-poly <vilib>:"FFT.vi"("X"=w761) -> ("FFT {X}"=w757:cdb[])  [unwired: 9 in, 1 out]
                    n249 = call-poly <vilib>:"FFT.vi"("X"=w765) -> ("FFT {X}"=w756:cdb[])  [unwired: 9 in, 1 out]
                    n250 = Index Array(array=w764, index (row)=0 ("索引"), index (col)=w758) -> (element=w759:i32)
                    n251 = Greater Than 0?(x=w759) -> (x > 0?=w755:bool)
                    n252 = case shown="假" w755 {
                      tunnel: w759 -> [w775 w777]
                      tunnel: w762 -> [w776 _]
                      tunnel: [w774 w777] -> w754
                      frame False {
                        n253 = Add(x=w776, y=w775) -> (x+y=w774:i32)
                      }
                      frame True {
                      }
                    }
                    n254 = Divide(x=w754, y=w763) -> (x/y=w753:dbl)
                    n255 = Index Array(array=w757, index=w753) -> (element=w751:cdb)
                    n256 = Index Array(array=w756, index=w753) -> (element=w750:cdb)
                    n257 = Subtract(x=w751, y=w748) -> (x-y=w747:cdb)
                    n258 = Subtract(x=w750, y=w749) -> (x-y=w746:cdb)
                  }
                }
                n259 = property on="小注入模式" class="DigNum (严格)"() -> ("Value"=w456:u8)  [unwired: 2 in, 2 out]
                n260 = property on="响应模式" class="DigNum (严格)"() -> ("Value"=w457:u8)  [unwired: 2 in, 2 out]
                n261 = Join Numbers(hi=w456, lo=w457) -> ((hi.lo)=w455:u16)
                n262 = Index Array(array=w451, index (row)=0 ("索引"), index (col)=w453) -> (element=w452:i32)
                n263 = case shown="769..771, 1281..1283" w455 {
                  tunnel: [w489 w504 w526 w527 w539] -> w476
                  tunnel: w472 -> [w489 w503 w525 w528 w540]
                  tunnel: w462 -> [_ w496 w515 w529 w541]
                  tunnel: w461 -> [_ _ _ w534 w550]
                  tunnel: w460 -> [_ w499 w519 _ _]
                  tunnel: w459 -> [_ w498 w518 w535 w552]
                  tunnel: w458 -> [_ _ w517 _ w551]
                  tunnel: w452 -> [_ w490 w505 _ _]
                  frame 0, Default {
                  }
                  frame 256, 512, 1024, 1536 {
                    # "自轴注入，自轴响应"
                    n264 = Divide(x=w498, y=w499) -> (x/y=w502:cdb)
                    n265 = Complex To Polar(r * e^(i*theta)=w502) -> (r=w493:dbl, theta=w501:dbl)
                    n266 = To Double Precision Float(number=w490) -> (double precision float=w491:dbl)
                    n267 = Multiply(x=w501, y=57.29577951308232) -> (x*y=w492:dbl)
                    n268 = Replace Array Subset(array=w503, new element #1=w491, index (row) #1=w496, index (col) #1=0, new element #2=w493, index (row) #2=w496, index (col) #2=1, new element #3=w492, index (row) #3=w496, index (col) #3=2) -> (w504:dbl[][])
                  }
                  frame 257..259, 513..515, 1025..1027, 1537..1539 {
                    w520 = 57.29577951308232
                    # "自轴注入，自、互轴响应"
                    n269 = Divide(x=w518, y=w519) -> (x/y=w524:cdb)
                    n270 = Divide(x=w517, y=w519) -> (x/y=w521:cdb)
                    n271 = Complex To Polar(r * e^(i*theta)=w524) -> (r=w510:dbl, theta=w523:dbl)
                    n272 = Complex To Polar(r * e^(i*theta)=w521) -> (r=w509:dbl, theta=w522:dbl)
                    n273 = To Double Precision Float(number=w505) -> (double precision float=w506:dbl)
                    n274 = Multiply(x=w523, y=w520) -> (x*y=w507:dbl)
                    n275 = Multiply(x=w522, y=w520) -> (x*y=w508:dbl)
                    n276 = Replace Array Subset(array=w525, new element #1=w506, index (row) #1=w515, index (col) #1=0, new element #2=w510, index (row) #2=w515, index (col) #2=1, new element #3=w507, index (row) #3=w515, index (col) #3=2, new element #4=w509, index (row) #4=w515, index (col) #4=3, new element #5=w508, index (row) #5=w515, index (col) #5=4) -> (w526:dbl[][])
                  }
                  frame 768, 1280 {
                    # "互轴注入，自轴响应"
                    n277 = Divide(x=w535, y=w534) -> (x/y=w538:cdb)
                    n278 = Complex To Polar(r * e^(i*theta)=w538) -> (r=w531:dbl, theta=w537:dbl)
                    n279 = Multiply(x=w537, y=57.29577951308232) -> (x*y=w533:dbl)
                    n280 = Replace Array Subset(array=w528, new element #1=w531, index (row) #1=w529, index (col) #1=5, new element #2=w533, index (row) #2=w529, index (col) #2=6) -> (w527:dbl[][])
                  }
                  frame 769..771, 1281..1283 {
                    w553 = 57.29577951308232
                    # "互轴注入，自、互轴响应"
                    n281 = Divide(x=w552, y=w550) -> (x/y=w557:cdb)
                    n282 = Divide(x=w551, y=w550) -> (x/y=w554:cdb)
                    n283 = Complex To Polar(r * e^(i*theta)=w557) -> (r=w543:dbl, theta=w556:dbl)
                    n284 = Complex To Polar(r * e^(i*theta)=w554) -> (r=w547:dbl, theta=w555:dbl)
                    n285 = Multiply(x=w556, y=w553) -> (x*y=w545:dbl)
                    n286 = Multiply(x=w555, y=w553) -> (x*y=w549:dbl)
                    n287 = Replace Array Subset(array=w540, new element #1=w543, index (row) #1=w541, index (col) #1=5, new element #2=w545, index (row) #2=w541, index (col) #2=6, new element #3=w547, index (row) #3=w541, index (col) #3=7, new element #4=w549, index (row) #4=w541, index (col) #4=8) -> (w539:dbl[][])
                  }
                }
              }
            }
          }
        }
        frame True {
          n288 = call-poly <vilib>:"FFT.vi"("X"=w790) -> ("FFT {X}"=w781:cdb[])  [unwired: 9 in, 1 out]
          n289 = call-poly <vilib>:"FFT.vi"("X"=w789) -> ("FFT {X}"=w780:cdb[])  [unwired: 9 in, 1 out]
          n290 = call-poly <vilib>:"FFT.vi"("X"=w782) -> ("FFT {X}"=w779:cdb[])  [unwired: 9 in, 1 out]
          n291 = for {
            tunnel: w788 -> [w807]
            tunnel: w787 -> [w802]
            tunnel: w786 -> [w801]
            tunnel: w781 -> [w799]
            tunnel: w780 -> [w798]
            tunnel: w779 -> [w797]
            shift-right: [w794] -> w783
            shift-left: w785 -> [w796]
            tunnel: w784 -> [w795] mode=indexing
            tunnel: w778 -> [w793]
            i -> [w792]
            n292 = Index Array(array=w807, index (row) #1=0 ("索引"), index (col) #1=w792, index (row) #2=1 ("索引"), index (col) #2=w792) -> (element #1=w803:i32, element #2=w800:i32)
            n293 = Index Array(array=w793, index (row)=w792) -> (element=w791:cdb[])  [unwired: 1 in]
            n294 = Not Equal To 0?(x=w803) -> (x != 0?=w804:bool)
            n295 = case shown="真" w804 {
              tunnel: w803 -> [_ w809]
              tunnel: w802 -> [_ w842]
              tunnel: w801 -> [_ w843]
              tunnel: w800 -> [_ w844]
              tunnel: w799 -> [_ w840]
              tunnel: w798 -> [_ w839]
              tunnel: w797 -> [_ w838]
              tunnel: w796 -> [w808 w835]
              tunnel: w795 -> [_ w834]
              tunnel: [w808 w833] -> w794
              tunnel: w791 -> [_ w831]
              frame False {
              }
              frame True {
                w815 = 57.29577951308232
                n296 = Greater Than 0?(x=w844) -> (x > 0?=w845:bool)
                n297 = Greater Than 0?(x=w809) -> (x > 0?=w847:bool)
                n298 = case shown="假" w847 {
                  tunnel: w809 -> [w853 w855]
                  tunnel: w843 -> [w854 _]
                  tunnel: [w852 w855] -> w846
                  frame False {
                    n299 = Add(x=w854, y=w853) -> (x+y=w852:i32)
                  }
                  frame True {
                  }
                }
                n300 = case shown="假" w845 {
                  tunnel: w844 -> [w849 w851]
                  tunnel: w843 -> [w850 _]
                  tunnel: [w848 w851] -> w841
                  frame False {
                    n301 = Add(x=w850, y=w849) -> (x+y=w848:i32)
                  }
                  frame True {
                  }
                }
                n302 = Index Array(array=w831, index #1=0 ("索引"), index #2=2 ("索引"), index #3=3 ("索引")) -> (element #1=w829:cdb, element #2=w823:cdb, element #3=w824:cdb)
                n303 = Divide(x=w846, y=w842) -> (x/y=w837:dbl)
                n304 = Divide(x=w841, y=w842) -> (x/y=w836:dbl)
                n305 = Index Array(array=w840, index=w837) -> (element=w830:cdb)
                n306 = Index Array(array=w839, index=w836) -> (element=w826:cdb)
                n307 = Index Array(array=w838, index=w836) -> (element=w825:cdb)
                n308 = Subtract(x=w830, y=w829) -> (x-y=w820:cdb)
                n309 = Subtract(x=w825, y=w824) -> (x-y=w821:cdb)
                n310 = Subtract(x=w826, y=w823) -> (x-y=w822:cdb)
                n311 = Divide(x=w822, y=w820) -> (x/y=w816:cdb)
                n312 = Divide(x=w821, y=w820) -> (x/y=w818:cdb)
                n313 = Complex To Polar(r * e^(i*theta)=w816) -> (r=w814:dbl, theta=w817:dbl)
                n314 = Complex To Polar(r * e^(i*theta)=w818) -> (r=w812:dbl, theta=w819:dbl)
                n315 = Multiply(x=w817, y=w815) -> (x*y=w813:dbl)
                n316 = Multiply(x=w819, y=w815) -> (x*y=w811:dbl)
                n317 = Build Array(w809, w814, w813, w812, w811) -> (w810:dbl[])
                n318 = Replace Array Subset(array=w835, new element=w810, index (row)=w834) -> (w833:dbl[][])  [unwired: 1 in]
              }
            }
          }
        }
      }
    }
    frame 100 {
      # "能测则测"
      n319 = case shown="1" "可用pico数(仅用于模式100)" {
        tunnel: [w870 w872 w935] -> w868
        tunnel: w869 -> [w870 w873 w936]
        tunnel: w865 -> [_ w874 w945]
        tunnel: w864 -> [_ w875 w944]
        tunnel: w863 -> [_ w871 _]
        tunnel: w862 -> [_ _ w943]
        tunnel: w861 -> [_ _ w942]
        tunnel: w860 -> [_ _ _]
        tunnel: w859 -> [_ w877 w941]
        tunnel: w858 -> [_ w876 w940]
        tunnel: w857 -> [_ w878 w939]
        tunnel: w856 -> [_ w879 w938]
        frame 0, Default {
        }
        frame 1 {
          n320 = call-poly <vilib>:"FFT.vi"("X"=w874) -> ("FFT {X}"=w882:cdb[])  [unwired: 9 in, 1 out]
          n321 = call-poly <vilib>:"FFT.vi"("X"=w875) -> ("FFT {X}"=w881:cdb[])  [unwired: 9 in, 1 out]
          n322 = call-poly <vilib>:"FFT.vi"("X"=w871) -> ("FFT {X}"=w880:cdb[])  [unwired: 9 in, 1 out]
          n323 = for {
            tunnel: w878 -> [w895]
            tunnel: w877 -> [w890]
            tunnel: w876 -> [w889]
            shift-right: [w886] -> w872
            shift-left: w873 -> [w888]
            tunnel: w879 -> [w887] mode=indexing
            tunnel: w882 -> [w885]
            tunnel: w881 -> [w884]
            tunnel: w880 -> [w883]
            i -> [w894]
            n324 = Index Array(array=w895, index (row)=0 ("索引"), index (col)=w894) -> (element=w891:i32)
            n325 = Not Equal To 0?(x=w891) -> (x != 0?=w892:bool)
            n326 = case shown="真" w892 {
              tunnel: w891 -> [_ w920]
              tunnel: w890 -> [_ w924]
              tunnel: w889 -> [_ w925]
              tunnel: w888 -> [w896 w923]
              tunnel: w887 -> [_ w921]
              tunnel: [w896 w922] -> w886
              tunnel: w885 -> [_ w915]
              tunnel: w884 -> [_ w919]
              tunnel: w883 -> [_ w917]
              frame False {
              }
              frame True {
                w897 = 0.0 ("元素")
                w899 = 57.29577951308232
                w898 = 2
                n327 = Greater Than 0?(x=w920) -> (x > 0?=w927:bool)
                n328 = case shown="假" w927 {
                  tunnel: w920 -> [w929 w931]
                  tunnel: w925 -> [w930 _]
                  tunnel: [w928 w931] -> w926
                  frame False {
                    n329 = Add(x=w930, y=w929) -> (x+y=w928:i32)
                  }
                  frame True {
                  }
                }
                n330 = Divide(x=w926, y=w924) -> (x/y=w916:dbl)
                n331 = Index Array(array=w915, index=w916) -> (element=w905:cdb)
                n332 = Index Array(array=w919, index=w916) -> (element=w904:cdb)
                n333 = Index Array(array=w917, index=w916) -> (element=w914:cdb)
                n334 = Complex To Polar(r * e^(i*theta)=w905) -> (r=w907:dbl, theta=w906:dbl)
                n335 = Complex To Polar(r * e^(i*theta)=w904) -> (r=w909:dbl, theta=w908:dbl)
                n336 = Complex To Polar(r * e^(i*theta)=w914) -> (r=w913:dbl, theta=w912:dbl)
                n337 = Multiply(x=w907, y=w898) -> (x*y=w900:dbl)
                n338 = Multiply(x=w909, y=w898) -> (x*y=w903:dbl)
                n339 = Multiply(x=w913, y=w898) -> (x*y=w911:dbl)
                n340 = Multiply(x=w906, y=w899) -> (x*y=w901:dbl)
                n341 = Multiply(x=w908, y=w899) -> (x*y=w902:dbl)
                n342 = Multiply(x=w912, y=w899) -> (x*y=w910:dbl)
                n343 = Build Array(w920, w900, w901, w903, w902, w911, w910, w897, w897) -> (w918:dbl[])
                n344 = Replace Array Subset(array=w923, new element=w918, index (row)=w921) -> (w922:dbl[][])  [unwired: 1 in]
              }
            }
          }
        }
        frame 2 {
          n345 = call-poly <vilib>:"FFT.vi"("X"=w945) -> ("FFT {X}"=w937:cdb[])  [unwired: 9 in, 1 out]
          n346 = call-poly <vilib>:"FFT.vi"("X"=w944) -> ("FFT {X}"=w934:cdb[])  [unwired: 9 in, 1 out]
          n347 = call-poly <vilib>:"FFT.vi"("X"=w943) -> ("FFT {X}"=w933:cdb[])  [unwired: 9 in, 1 out]
          n348 = call-poly <vilib>:"FFT.vi"("X"=w942) -> ("FFT {X}"=w932:cdb[])  [unwired: 9 in, 1 out]
          n349 = for {
            tunnel: w939 -> [w959]
            tunnel: w941 -> [w954]
            tunnel: w940 -> [w953]
            shift-right: [w950] -> w935
            shift-left: w936 -> [w952]
            tunnel: w938 -> [w951] mode=indexing
            tunnel: w937 -> [w949]
            tunnel: w934 -> [w948]
            tunnel: w933 -> [w947]
            tunnel: w932 -> [w946]
            i -> [w958]
            n350 = Index Array(array=w959, index (row)=0 ("索引"), index (col)=w958) -> (element=w955:i32)
            n351 = Not Equal To 0?(x=w955) -> (x != 0?=w956:bool)
            n352 = case shown="真" w956 {
              tunnel: w955 -> [_ w989]
              tunnel: w954 -> [_ w993]
              tunnel: w953 -> [_ w994]
              tunnel: w952 -> [w960 w992]
              tunnel: w951 -> [_ w990]
              tunnel: [w960 w991] -> w950
              tunnel: w949 -> [_ w979]
              tunnel: w948 -> [_ w988]
              tunnel: w947 -> [_ w985]
              tunnel: w946 -> [_ w986]
              frame False {
              }
              frame True {
                w962 = 57.29577951308232
                w961 = 2
                n353 = Greater Than 0?(x=w989) -> (x > 0?=w996:bool)
                n354 = case shown="假" w996 {
                  tunnel: w989 -> [w998 w1000]
                  tunnel: w994 -> [w999 _]
                  tunnel: [w997 w1000] -> w995
                  frame False {
                    n355 = Add(x=w999, y=w998) -> (x+y=w997:i32)
                  }
                  frame True {
                  }
                }
                n356 = Divide(x=w995, y=w993) -> (x/y=w984:dbl)
                n357 = Index Array(array=w979, index=w984) -> (element=w968:cdb)
                n358 = Index Array(array=w988, index=w984) -> (element=w967:cdb)
                n359 = Index Array(array=w985, index=w984) -> (element=w977:cdb)
                n360 = Index Array(array=w986, index=w984) -> (element=w978:cdb)
                n361 = Complex To Polar(r * e^(i*theta)=w968) -> (r=w970:dbl, theta=w969:dbl)
                n362 = Complex To Polar(r * e^(i*theta)=w967) -> (r=w972:dbl, theta=w971:dbl)
                n363 = Complex To Polar(r * e^(i*theta)=w977) -> (r=w976:dbl, theta=w975:dbl)
                n364 = Complex To Polar(r * e^(i*theta)=w978) -> (r=w983:dbl, theta=w982:dbl)
                n365 = Multiply(x=w970, y=w961) -> (x*y=w963:dbl)
                n366 = Multiply(x=w972, y=w961) -> (x*y=w966:dbl)
                n367 = Multiply(x=w976, y=w961) -> (x*y=w974:dbl)
                n368 = Multiply(x=w983, y=w961) -> (x*y=w980:dbl)
                n369 = Multiply(x=w969, y=w962) -> (x*y=w964:dbl)
                n370 = Multiply(x=w971, y=w962) -> (x*y=w965:dbl)
                n371 = Multiply(x=w975, y=w962) -> (x*y=w973:dbl)
                n372 = Multiply(x=w982, y=w962) -> (x*y=w981:dbl)
                n373 = Build Array(w989, w963, w964, w966, w965, w974, w973, w980, w981) -> (w987:dbl[])
                n374 = Replace Array Subset(array=w992, new element=w987, index (row)=w990) -> (w991:dbl[][])  [unwired: 1 in]
              }
            }
          }
        }
      }
    }
  }
  "稳态工作点输出" <- w25
  "写表结果输出" <- w24
